vi "mod_scale number.vi"(1 "Ctrl Reference":refnum<vi>, 2 "number with scale":T1 {"scale" items=["T", "G", "M", "k", "", "m", "u", "n", "p", "f", "a"]; "number" format="%.2f"}) -> (0 "scaled number":dbl format="%.2p")   [LabVIEW 2020, in "niAMT.lvlib"]
uses:
  <vilib>/addons/Modulation/niAMT.lvlib
  <vilib>/addons/Modulation/Analog/controls/mod_Scaled Number.ctl
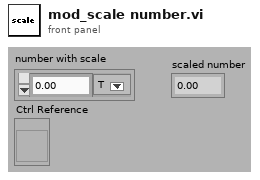
[diagram p1: front panel]
types:
  T1 = typedef "niAMT.lvlib/mod_Scaled Number.ctl" = cluster{"number":dbl, "scale":i32}
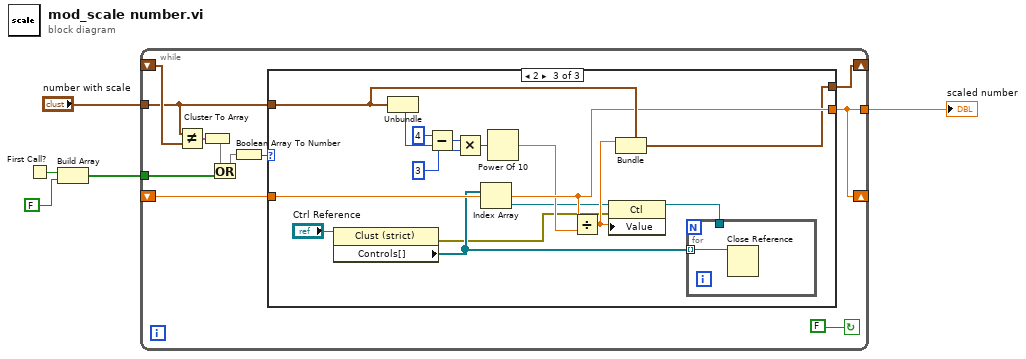
[diagram p0: block diagram]
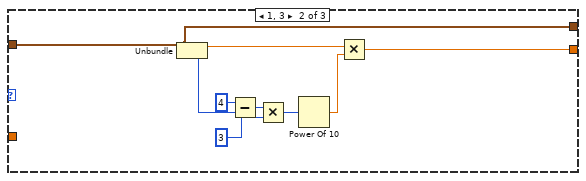
[diagram p3: hidden frame]
diagram:
  n1 = First Call?() -> (First Call?: T/F=w3:bool)
  n2 = Build Array(w3, FALSE ("element")) -> (w1:bool[])
  n3 = while {
    tunnel: "number with scale" -> [w7]
    tunnel: [w12] -> w4
    shift-right: [w6] -> _
    shift-left: _ -> [w8]
    shift-right: [w12] -> _
    shift-left: _ -> [w9]
    tunnel: w1 -> [w10]
    stop <- FALSE continue-if-true
    n4 = Not Equal?(x=w7, y=w8) -> (x != y?=w15:cluster{"number":bool, "scale":bool})
    n5 = Cluster To Array(cluster=w15) -> (array=w14:bool[])
    n6 = Or(x=w14, y=w10) -> (x .or. y?=w11:bool[])
    n7 = Boolean Array To Number(Boolean array=w11) -> (number=w13:u32)
    n8 = case shown="2" w13 {
      tunnel: [w18 w27 w36] -> w12
      tunnel: w7 -> [w17 w19 w42]
      tunnel: w9 -> [w18 _ w36]
      tunnel: [w17 w19 w34] -> w6
      frame 0, Default {
      }
      frame 1, 3 {
        n9 = Unbundle(w19) -> ("number"=w21:dbl, "scale"=w20:i32)
        n10 = Subtract(x=4, y=w20) -> (x-y=w25:i32)
        n11 = Multiply(x=w25, y=3) -> (x*y=w23:i32)
        n12 = Power Of 10(x=w23) -> (10^x=w22:dbl)
        n13 = Multiply(x=w21, y=w22) -> (x*y=w27:dbl)
      }
      frame 2 {
        n14 = property class="Clust (strict)"(reference="Ctrl Reference") -> (error out=w28:errorcluster, "Controls[]"=w32:refnum<vi>[])  [unwired: 1 in, 1 out]
        n15 = Unbundle(w42) -> ("scale"=w29:i32)  [unwired: 1 out]
        n16 = Subtract(x=4, y=w29) -> (x-y=w40:i32)
        n17 = Multiply(x=w40, y=3) -> (x*y=w38:i32)
        n18 = Index Array(array=w32) -> (element=w30:refnum<vi>)  [unwired: 1 in]
        n19 = Power Of 10(x=w38) -> (10^x=w35:dbl)
        n20 = Divide(x=w36, y=w35) -> (x/y=w37:dbl)
        n21 = property class="Ctl"(reference=w30, error in=w28, "Value"=w37) -> (reference out=w31:refnum<vi>)  [unwired: 1 out]
        n22 = Bundle(cluster=w42, "number"=w37) -> (w34:T1)  [unwired: 1 out]
        n23 = for {
          tunnel: w32 -> [w43] mode=indexing
          tunnel: w31 -> [_]
          n24 = Close Reference(reference=w43) -> ()  [unwired: 1 in, 1 out]
        }
      }
    }
  }
  "scaled number" <- w4
